vi "动力环境监测系统.vi"() -> ()   [LabVIEW 2016, in "环境动力监测库.lvlib"]
panel:
  in  "单选按钮":enum32{"首页", "设备配置"}(radio)
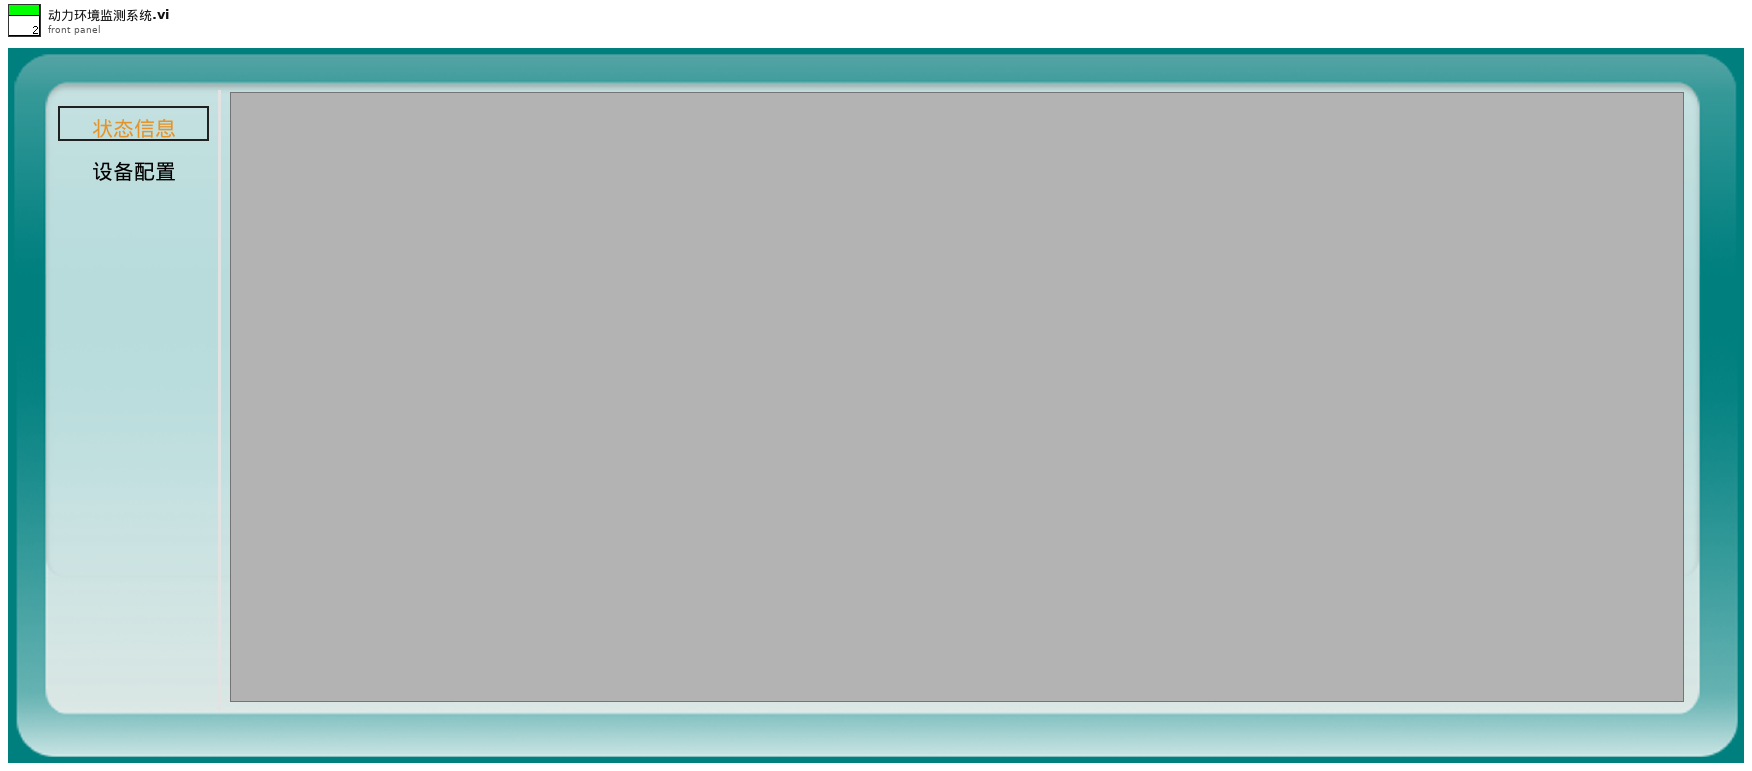
[diagram p1: front panel]
types:
  T1 = enum32{"Bad", "Idle", "Run top level", "Running"}
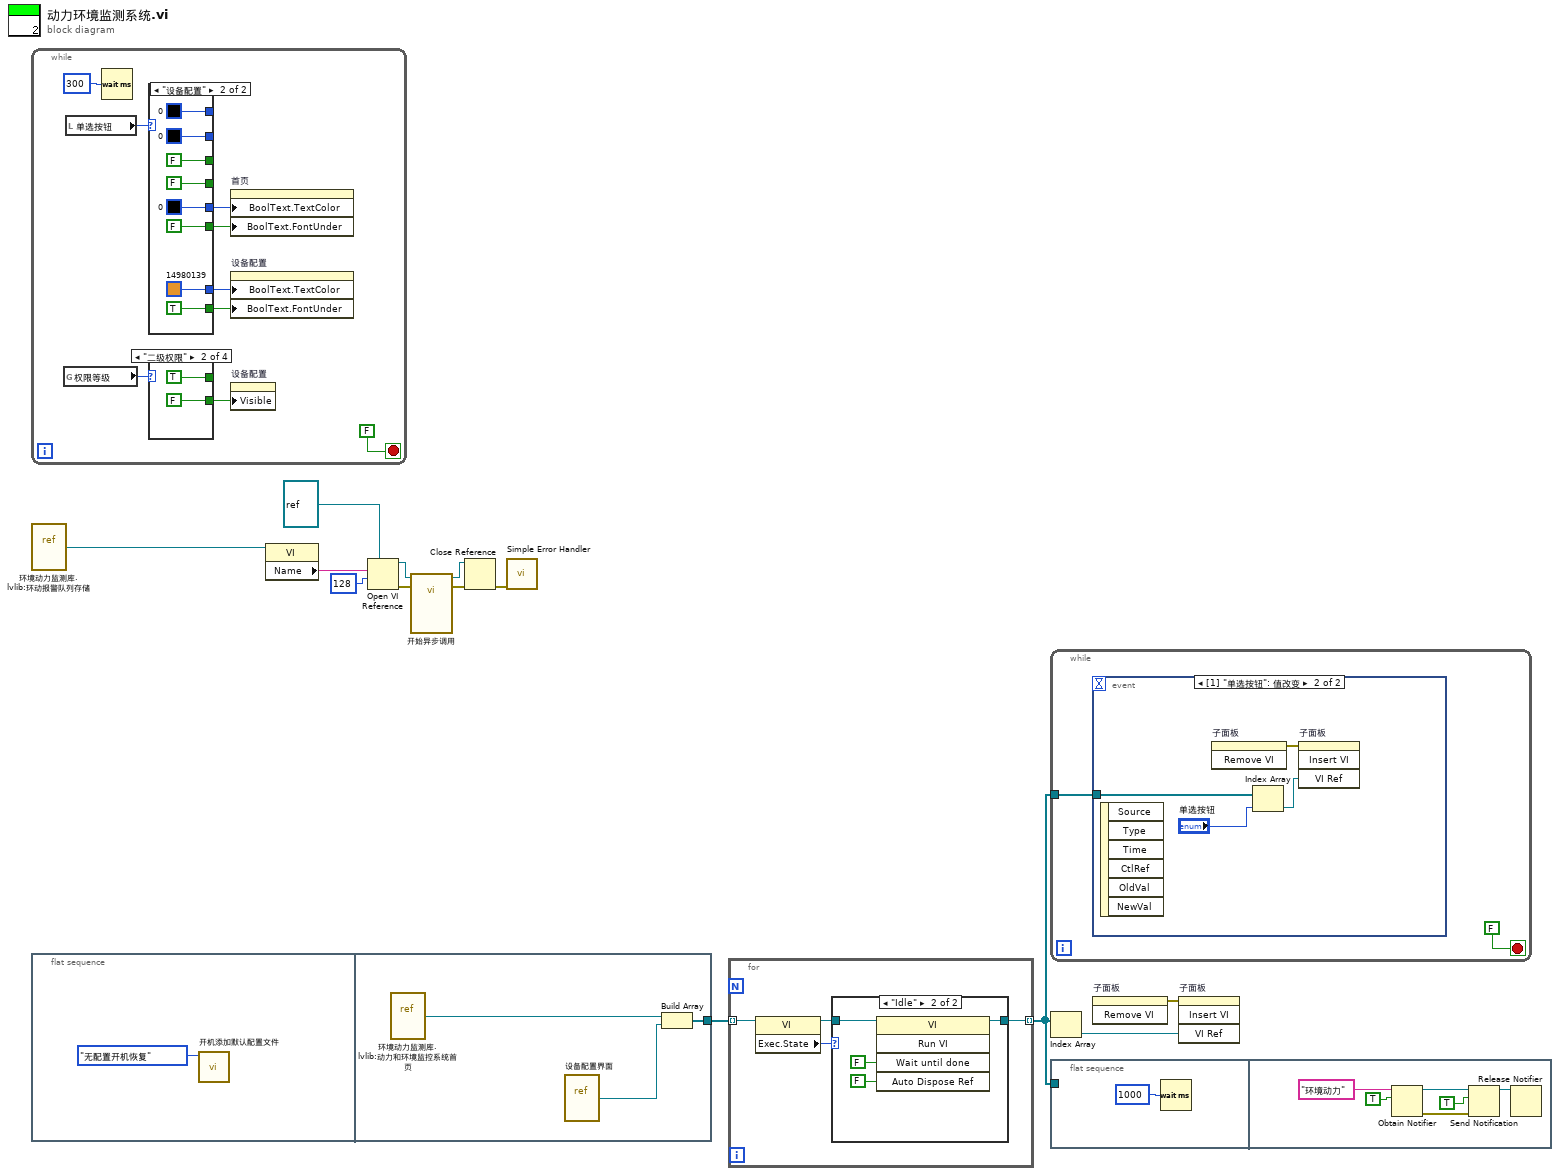
[diagram p0: block diagram]
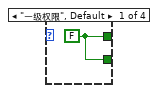
[diagram p2: hidden frame]
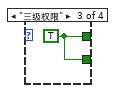
[diagram p3: hidden frame]
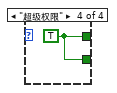
[diagram p4: hidden frame]
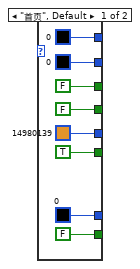
[diagram p5: hidden frame]
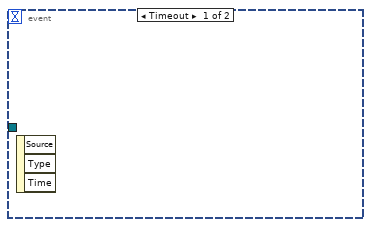
[diagram p6: hidden frame]
diagram:
  n1 = while {
    stop <- FALSE stop-if-true
    n2 = global read "外部交互全局变量.vi" "权限等级"() -> (w15:enum16{"一级权限", "二级权限", "三级权限", "超级权限"})
    n3 = local read "单选按钮"() -> (w18:enum32{"首页", "设备配置"})
    n4 = Wait (ms)(milliseconds to wait=u32 300 ("等待时间（毫秒）")) -> ()  [unwired: 1 out]
    n5 = case shown="\"设备配置\"" w18 {
      tunnel: [u32 0 u32 14980139] -> w21
      tunnel: [FALSE ("布尔文本.字体:下划线") TRUE ("布尔文本.字体:下划线")] -> w22
      tunnel: [u32 0 u32 0] -> _
      tunnel: [FALSE ("布尔文本.字体:下划线") FALSE ("布尔文本.字体:下划线")] -> _
      tunnel: [u32 14980139 u32 0] -> w19
      tunnel: [TRUE ("布尔文本.字体:下划线") FALSE ("布尔文本.字体:下划线")] -> w20
      tunnel: [u32 0 u32 0] -> _
      tunnel: [FALSE ("布尔文本.字体:下划线") FALSE ("布尔文本.字体:下划线")] -> _
      frame "首页", Default {
      }
      frame "设备配置" {
      }
    }
    n6 = case shown="\"二级权限\"" w15 {
      tunnel: [w23 TRUE w26 w27] -> _
      tunnel: [w23 FALSE w26 w27] -> w14
      frame "一级权限", Default {
        w23 = FALSE
      }
      frame "二级权限" {
      }
      frame "三级权限" {
        w26 = TRUE
      }
      frame "超级权限" {
        w27 = TRUE
      }
    }
    n7 = property on="首页" class="Bool (严格)"("BoolText.TextColor"=w19, "BoolText.FontUnder"=w20) -> ()  [unwired: 2 in, 2 out]
    n8 = property on="设备配置" class="Bool (严格)"("BoolText.TextColor"=w21, "BoolText.FontUnder"=w22) -> ()  [unwired: 2 in, 2 out]
    n9 = property on="设备配置" class="Bool (严格)"("Visible"=w14) -> ()  [unwired: 2 in, 2 out]
  }
  n10 = vi-ref "环境动力监测库.lvlib:环动报警队列存储.vi"() -> (w8:refnum<vi>)
  n11 = flat-sequence {
    tunnel: [w47] -> w13
    frame #0 {
      n12 = call "开机添加默认配置文件.vi"("恢复默认方式"=enum16{"无配置开机恢复", "手动恢复"}."无配置开机恢复") -> ()  [unwired: 10 in, 1 out]
    }
    frame #1 {
      n13 = vi-ref "环境动力监测库.lvlib:动力和环境监控系统首页.vi"() -> (w45:refnum<vi>)
      n14 = vi-ref "设备配置界面.vi"() -> (w46:refnum<vi>)
      n15 = Build Array(w45, w46) -> (w47:refnum<vi>[])
    }
  }
  n16 = property class="VI"(reference=w8) -> ("Name"=w7:string)  [unwired: 1 in, 2 out]
  n17 = Open VI Reference(type specifier VI Refnum (for type only)=refnum<vi> refnum ("类型说明符VI引用句柄（仅用于类型）"), vi path=w7, options=128 ("选项")) -> (vi reference=w5:refnum<vi>, error out=w9:errorcluster)  [unwired: 3 in]
  n18 = call-by-ref "开始异步调用"(reference=w5, error in=w9) -> (reference out=w4:refnum<vi>, error out=w3:errorcluster)  [unwired: 12 in]
  n19 = Close Reference(reference=w4, error in (no error)=w3) -> (error out=w2:errorcluster)
  n20 = call <vilib>:"Simple Error Handler.vi"("error in (no error)"=w2) -> ()  [unwired: 4 in, 5 out]
  n21 = for {
    tunnel: w13 -> [w51] mode=indexing
    tunnel: [w50] -> w1 mode=indexing
    n22 = property class="VI"(reference=w51) -> (reference out=w48:refnum<vi>, "Exec.State"=w49:T1)  [unwired: 1 in, 1 out]
    n23 = case shown="\"Idle\"" w49 {
      tunnel: w48 -> [w52 w54]
      tunnel: [w52 w53] -> w50
      frame "Bad", Default {
      }
      frame "Idle" {
        n24 = invoke class="VI" method="Run VI"(reference=w54, "Wait until done"=FALSE ("结束前等待"), "Auto Dispose Ref"=FALSE ("自动销毁引用")) -> (reference out=w53:refnum<vi>)  [unwired: 2 in, 4 out]
      }
    }
  }
  n25 = while {
    tunnel: w1 -> [w57]
    stop <- FALSE stop-if-true
    n26 = event shown="[1] \"单选按钮\": 值改变" {
      selector: _ -> [_ _]
      dyn-events: _ -> [_ _]
      timeout: _ -> [_ _]
      tunnel: w57 -> [_ w60]
      event Timeout {
        n27 = event-data() -> ()  [unwired: 1 in, 3 out]
      }
      event "单选按钮": Value Change {
        n28 = event-data() -> ()  [unwired: 1 in, 6 out]
        n29 = invoke on="子面板" class="SubPnl" method="Remove VI"() -> (error out=w62:errorcluster)  [unwired: 3 in, 2 out]
        n30 = Index Array(array=w60, index="单选按钮") -> (element=w61:refnum<vi>)
        n31 = invoke on="子面板" class="SubPnl" method="Insert VI"(error in=w62, "VI Ref"=w61) -> ()  [unwired: 2 in, 4 out]
      }
    }
  }
  n32 = Index Array(array=w1) -> (element=w11:refnum<vi>)  [unwired: 1 in]
  n33 = flat-sequence {
    tunnel: w1 -> [_]
    frame #0 {
      n34 = Wait (ms)(milliseconds to wait=u32 1000 ("等待时间（毫秒）")) -> ()  [unwired: 1 out]
    }
    frame #1 {
      n35 = Obtain Notifier(name (unnamed)="环境动力" ("名称（未命名）"), notification data type=TRUE) -> (notifier out=w68:refnum<notifier>, error out=w64:errorcluster)  [unwired: 2 in, 1 out]
      n36 = Send Notification(notification=TRUE ("通知"), notifier=w68, error in (no error)=w64) -> (notifier out=w67:refnum<notifier>)  [unwired: 1 out]
      n37 = Release Notifier(notifier=w67) -> ()  [unwired: 2 in, 3 out]
    }
  }
  n38 = invoke on="子面板" class="SubPnl" method="Remove VI"() -> (error out=w12:errorcluster)  [unwired: 3 in, 2 out]
  n39 = invoke on="子面板" class="SubPnl" method="Insert VI"(error in=w12, "VI Ref"=w11) -> ()  [unwired: 2 in, 4 out]
